vi "AVI-video length info.vi"(8 "error in (no error)":errorcluster) -> (0 "error out":errorcluster, 1 "Expected number of speed values":dbl, 3 "Video length info":string)   [LabVIEW 2013]
uses:
  Globals/gl_Time series viewer globals.vi
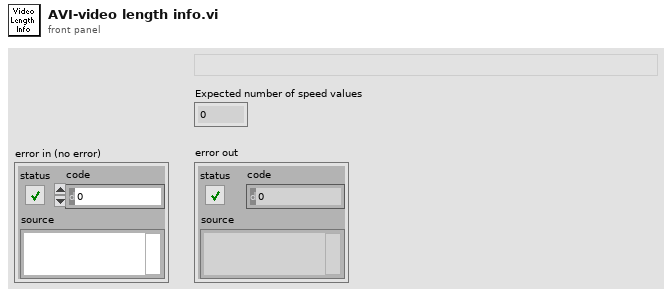
[diagram p1: front panel]
types:
  T1 = typedef "Timelapse viewer refs.ctl" = cluster{"This VI":refnum<vi>, "AVI Mode ind":refnum<vi>, "Play":refnum<vi>, "Stop":refnum<vi>, "Back":refnum<vi>, "Scrollbar":refnum<vi>, "Video length info":refnum<vi>, "Expected speed values":refnum<vi>, "Intensity":refnum<vi>, "Path":refnum<vi>, "Selection sliders":refnum<vi>, "Speed Graph ref":refnum<vi>, "Frame rate set (fps)":refnum<vi>}
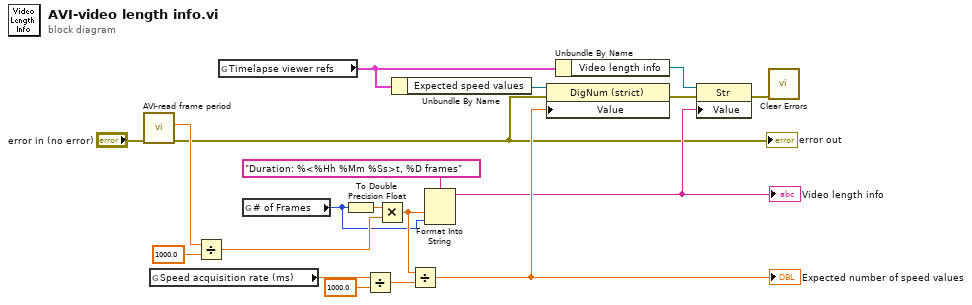
[diagram p0: block diagram]
diagram:
  n1 = call "AVI-read frame period.vi"("error in (no error)"="error in (no error)") -> ("error out"=w2:errorcluster, "Frame period (ms)"=w15:dbl)  [unwired: 9 in]
  "error out" <- w2
  n2 = global read "gl_Time series viewer globals.vi" "Speed acquisition rate (ms)"() -> (w11:dbl)
  n3 = Divide(x=w15, y=1000.0) -> (x/y=w17:dbl)
  n4 = global read "gl_Time series viewer globals.vi" "Timelapse viewer refs"() -> (w9:T1)
  n5 = global read "gl_Time series viewer globals.vi" "# of Frames"() -> (w3:u32)
  n6 = To Double Precision Float(number=w3) -> (double precision float=w18:dbl)
  n7 = Divide(x=w11, y=1000.0) -> (x/y=w13:dbl)
  n8 = Multiply(x=w18, y=w17) -> (x*y=w4:dbl)
  n9 = Unbundle By Name(w9) -> ("Expected speed values"=w10:refnum<vi>)
  n10 = Divide(x=w4, y=w13) -> (x/y=w8:dbl)
  "Expected number of speed values" <- w8
  n11 = Format Into String(format string="Duration: %<%Hh %Mm %Ss>t, %D frames", w4, w3) -> (resulting string=w6:string)  [unwired: 2 in, 1 out]
  "Video length info" <- w6
  n12 = property class="DigNum (strict)"(reference=w10, error in=w2, "Value"=w8) -> (error out=w7:errorcluster)  [unwired: 1 out]
  n13 = Unbundle By Name(w9) -> ("Video length info"=w5:refnum<vi>)
  n14 = property class="Str"(reference=w5, error in=w7, "Value"=w6) -> (error out=w1:errorcluster)  [unwired: 1 out]
  n15 = call <vilib>:"Clear Errors.vi"("error in (no error)"=w1) -> ()  [unwired: 6 in, 1 out]
